vi "monitoring Screen 2.vi"() -> ()   [LabVIEW 2022 SP3]
panel:
  out "V_AB":dbl caption="A-Phase ATF" format="%#_6g.00K"
  out "I_C":dbl caption="A-Phase ATF" format="%#_6g.00A"
  out "I_B":dbl caption="A-Phase ATF" format="%#_6g.00A"
  out "I_A":dbl caption="A-Phase ATF" format="%#_6g.00A"
  out "V_CA":dbl caption="A-Phase ATF" format="%#_6g.00V"
  out "V_BC":dbl caption="A-Phase ATF" format="%#_6g.00V"
  out "MW_3":dbl caption="A-Phase ATF" format="%#_6g.00K"
  out "MW_2":dbl caption="A-Phase ATF" format="%#_6g.00K"
  out "MW_1":dbl caption="A-Phase ATF" format="%#_6g.00K"
  out "C-Phase":dbl caption="A-Phase ATF" format="%#_6g.00K"
  out "B-Phase":dbl caption="A-Phase ATF" format="%#_6g.00K"
  out "A-Phase":dbl caption="A-Phase ATF" format="%#_6g.00K"
  out "Sector":dbl caption="A-Phase ATF" format="%#_6g.00"
  out "Run_duty_ratio":dbl caption="A-Phase ATF" format="%#_6g.00"
  out "Speed":dbl caption="A-Phase ATF" format="%#_6g.00 r/m"
  out "Voltage_Speed":dbl caption="A-Phase ATF" format="%#_6g.00 r/m"
  out "Speed":dbl caption="A-Phase ATF" format="%#_6g.00 r/m"
  out "Voltage_Speed":dbl caption="A-Phase ATF" format="%#_6g.00 r/m"
  out "Sector":dbl caption="A-Phase ATF" format="%#_6g.00"
  out "Run_duty_ratio":dbl caption="A-Phase ATF" format="%#_6g.00"
  out "Run ACK":bool
  out "M_State":bool
  out "Run ACK":bool
  out "M_State":bool
  out "FM_3":dbl caption="A-Phase ATF" format="%#_6g.00kg/s"
  out "FM_1":dbl caption="A-Phase ATF" format="%#_6g.00kg/s"
  out "FM_2":dbl caption="A-Phase ATF" format="%#_6g.00kg/s"
  out "Motor _NDE":dbl caption="A-Phase ATF" format="%#_6g.00"
  out "Motor_DE":dbl caption="A-Phase ATF" format="%#_6g.00"
  out "Motor_Casing":dbl caption="A-Phase ATF" format="%#_6g.00"
  out "I_DC":dbl caption="A-Phase ATF" format="%#_6g.00A"
  out "I_DC":dbl caption="A-Phase ATF" format="%#_6g.00A"
  out "V_DC":dbl caption="A-Phase ATF" format="%#_6g.00V"
  out "V_DC":dbl caption="A-Phase ATF" format="%#_6g.00V"
  out "I_DC":dbl caption="A-Phase ATF" format="%#_6g.00A"
  out "I_DC":dbl caption="A-Phase ATF" format="%#_6g.00A"
  out "V_DC":dbl caption="A-Phase ATF" format="%#_6g.00V"
  out "V_DC":dbl caption="A-Phase ATF" format="%#_6g.00V"
  out "FM_3":dbl caption="A-Phase ATF" format="%#_6g.00kg/s"
  out "FM_1":dbl caption="A-Phase ATF" format="%#_6g.00kg/s"
  out "FM_2":dbl caption="A-Phase ATF" format="%#_6g.00kg/s"
  out "Motor _NDE":dbl caption="A-Phase ATF" format="%#_6g.00"
  out "Motor_DE":dbl caption="A-Phase ATF" format="%#_6g.00"
  out "Motor_Casing":dbl caption="A-Phase ATF" format="%#_6g.00"
  out "U_AT_P_19":dbl caption="A-Phase ATF" format="%#_6g.00bar"
  out "U_EV_P_04":dbl caption="A-Phase ATF" format="%#_6g.00bar"
  out "U_LO_P_28":dbl caption="A-Phase ATF" format="%#_6g.00bar"
  out "U_EV_P_03       2":dbl caption="A-Phase ATF" format="%#_6g.00bar"
  out "U_EV_P_06":dbl caption="A-Phase ATF" format="%#_6g.00bar"
  out "U_EV_P_02":dbl caption="A-Phase ATF" format="%#_6g.00bar"
  out "U_EV_P_05":dbl caption="A-Phase ATF" format="%#_6g.00bar"
  out "U_EV_P_01":dbl caption="A-Phase ATF" format="%#_6g.00bar"
  out "U_AT_T_07":dbl caption="A-Phase ATF" format="%#_6g.00K"
  out "U_LO_T_18":dbl caption="A-Phase ATF" format="%#_6g.00K"
  out "U_EV_P_01":dbl caption="A-Phase ATF" format="%#_6g.00K"
  out "U_EV_P_01":dbl caption="A-Phase ATF" format="%#_6g.00K"
  out "U_EV_P_01":dbl caption="A-Phase ATF" format="%#_6g.00K"
  out "U_EV_P_01":dbl caption="A-Phase ATF" format="%#_6g.00K"
  out "U_EV_P_01":dbl caption="A-Phase ATF" format="%#_6g.00K"
  out "U_EV_P_01":dbl caption="A-Phase ATF" format="%#_6g.00K"
  out "U_EV_P_01":dbl caption="A-Phase ATF" format="%#_6g.00K"
  out "U_EV_P_01":dbl caption="A-Phase ATF" format="%#_6g.00K"
  out "E_Surface_RTD":dbl caption="A-Phase ATF" format="%#_6g.00K"
  out "Bearing_RTD":dbl caption="A-Phase ATF" format="%#_6g.00K"
  out "LC_Y":dbl caption="A-Phase ATF" format="%#_6g.00N"
  out "LC_Z":dbl caption="A-Phase ATF" format="%#_6g.00N"
  out "LC_X":dbl caption="A-Phase ATF" format="%#_6g.00N"
  out "RTD 5":dbl caption="A-Phase ATF" format="%#_6g.00K"
  out "RTD 6":dbl caption="A-Phase ATF" format="%#_6g.00K"
  out "RTD 7":dbl caption="A-Phase ATF" format="%#_6g.00K"
  out "RTD 8":dbl caption="A-Phase ATF" format="%#_6g.00K"
  out "RTD 1":dbl caption="A-Phase ATF" format="%#_6g.00K"
  out "RTD 2":dbl caption="A-Phase ATF" format="%#_6g.00K"
  out "RTD 3":dbl format="%#_6g.00K"
  out "RTD 4":dbl caption="A-Phase ATF" format="%#_6g.00K"
  out "V_AB":dbl caption="A-Phase ATF" format="%#_6g.00K"
  out "I_C":dbl caption="A-Phase ATF" format="%#_6g.00A"
  out "I_B":dbl caption="A-Phase ATF" format="%#_6g.00A"
  out "I_A":dbl caption="A-Phase ATF" format="%#_6g.00A"
  out "V_CA":dbl caption="A-Phase ATF" format="%#_6g.00V"
  out "V_BC":dbl caption="A-Phase ATF" format="%#_6g.00V"
  out "MW_3":dbl caption="A-Phase ATF" format="%#_6g.00K"
  out "MW_ 2":dbl caption="A-Phase ATF" format="%#_6g.00K"
  out "MW_1":dbl caption="A-Phase ATF" format="%#_6g.00K"
  out "C-Phase":dbl caption="A-Phase ATF" format="%#_6g.00K"
  out "B-Phase":dbl caption="A-Phase ATF" format="%#_6g.00K"
  out "A-Phase":dbl caption="A-Phase ATF" format="%#_6g.00K"
  out "SYNC":bool
  out "UDP":bool
  out "Log":bool
  out "PXI":bool
  in  "Screen No":dbl
  in  "Power 2":bool
  out "COUNT DOWN TIMER":dbl format="T%<+%H:%M:%S%3u>t"
  # "Agnite Engine Monitoring Screen"
  # "VERSION 1.3"
  # "ATF Drive Parameters"
  # "LOX Drive Parameters"
  # "Engine"
  # "Motor Run Speed"
  # "ATF Drive"
  # "Motor Run Speed"
  # "25000"
  # "rpm"
  # "25000"
  # "rpm"
  # "332"
  # "Hz"
  # "332"
  # "Hz"
  # "Voltage"
  # "Current"
  # "Flow Rate"
  # "Motor Temperature"
  # "Current"
  # "Voltage"
  # "Flow Rate"
  # "Motor Temperature"
  # "Pressure"
  # "Temperature"
  # "Health Status"
  # "Name: Vishali S"
  # "Data:01/11/2025"
  # "G N I K U L"
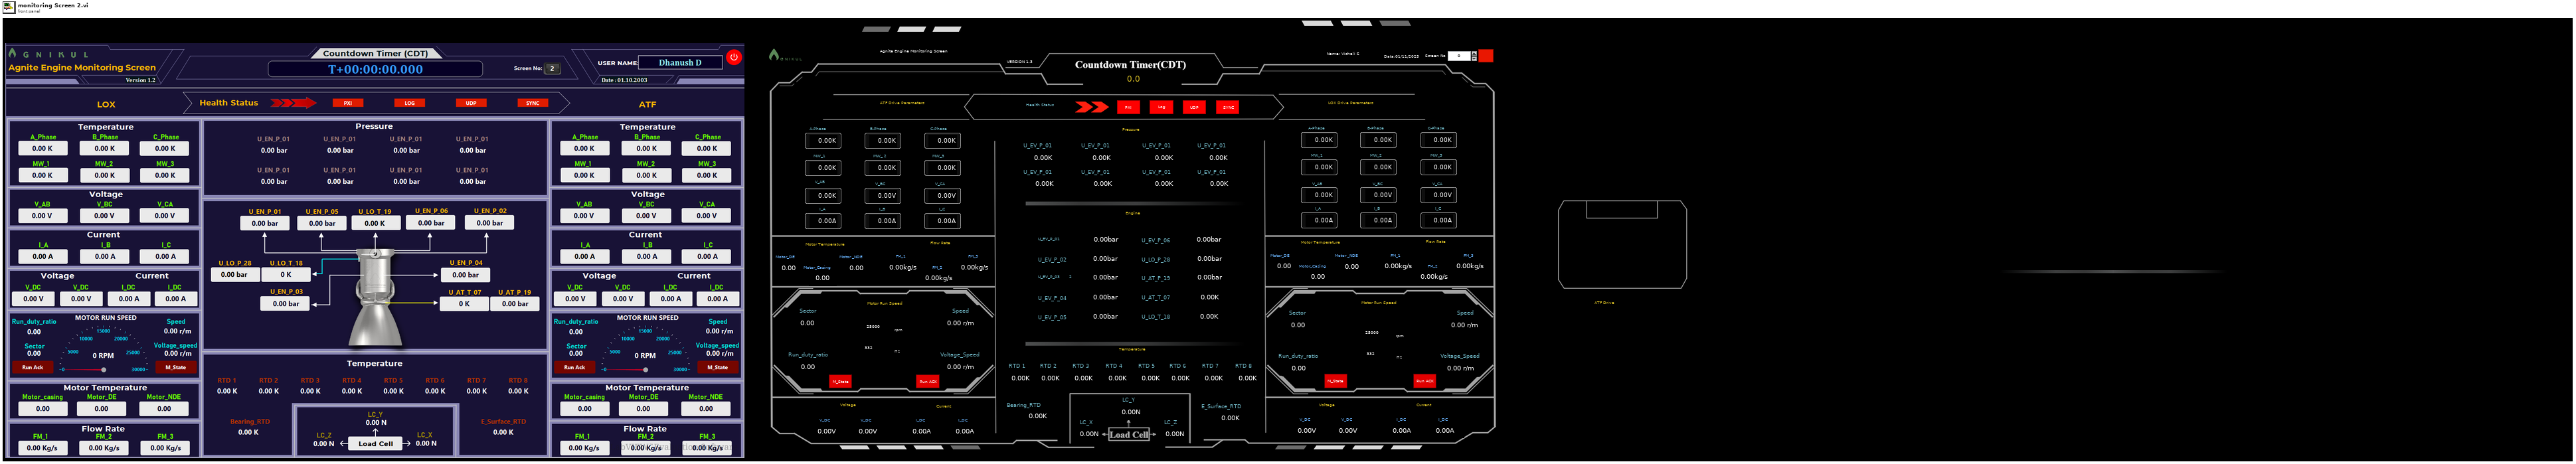
[diagram p1: front panel]
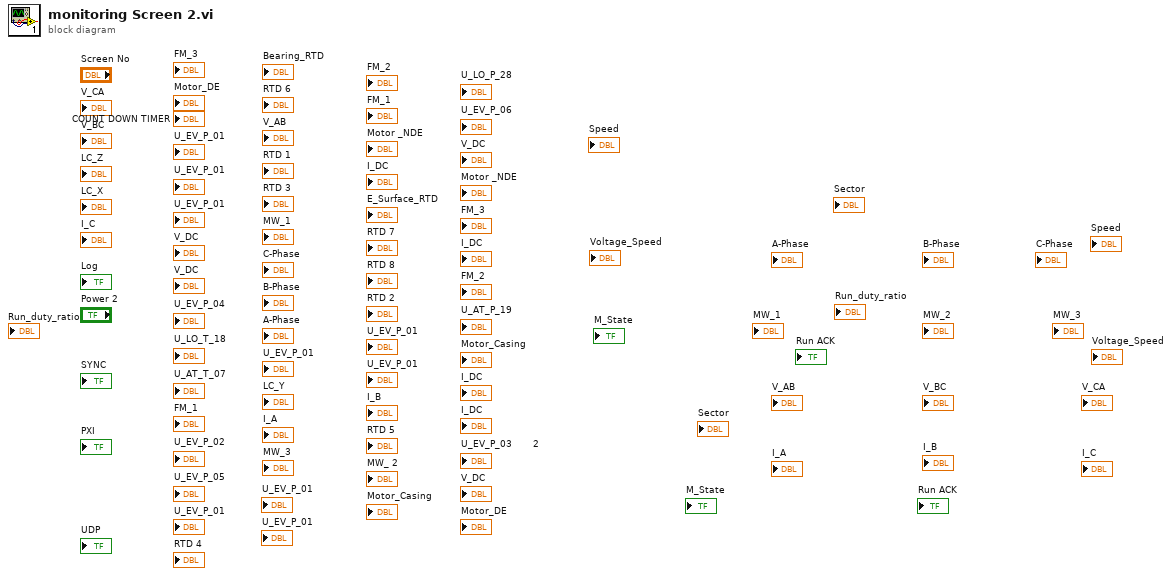
[diagram p0: block diagram]
diagram:
